vi "AO Post Step Type.vi"(8 "error in (no error)":errorcluster, 9 "AOWrite":T1, 10 "Socket No":u16=1, 11 "AO in":refnum<class "AO.lvclass">) -> (0 "error out":errorcluster, 2 "PhysicalChannel":string[](array[string]), 3 "AO out":refnum<class "AO.lvclass">)   [LabVIEW 2023, in "HardwareAbstractionLayer_LVOOP.lvlib" / "AO.lvclass"]
uses:
  AO.lvclass
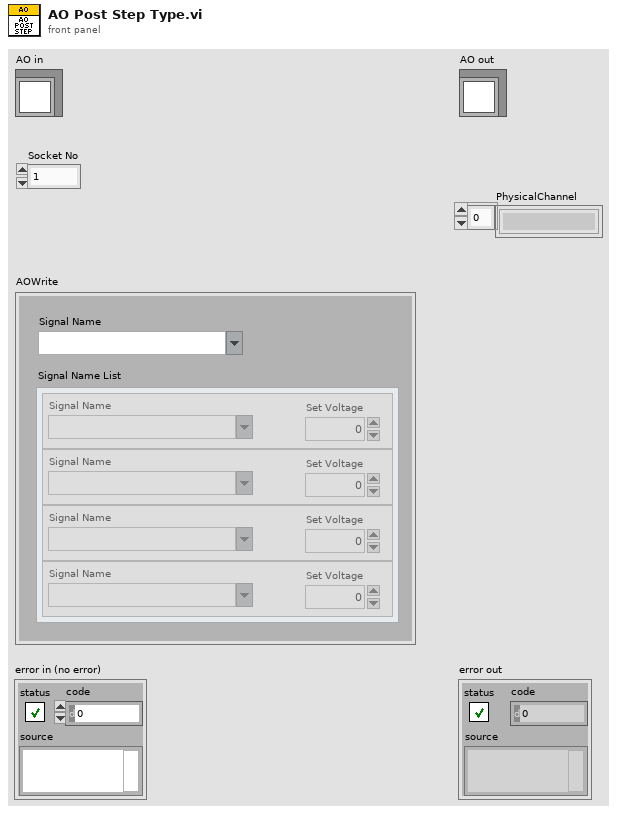
[diagram p1: front panel]
types:
  T1 = cluster{"Signal Name":string, "Signal Name List":cluster{"Signal Name":string, "Set Voltage":dbl}[]}
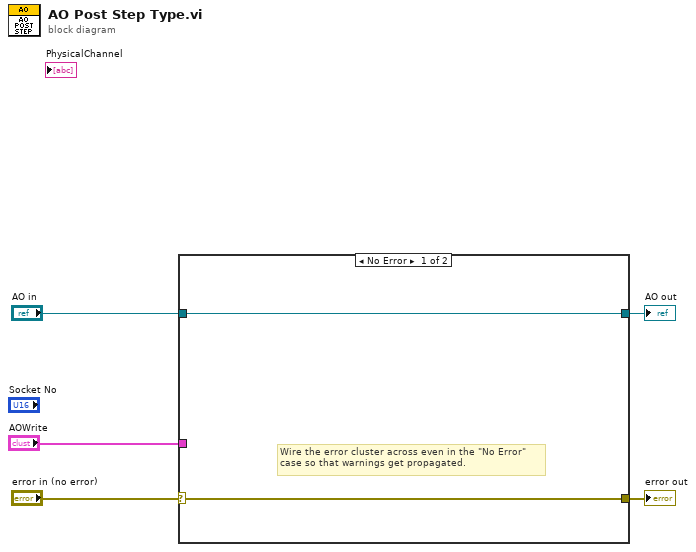
[diagram p0: block diagram]
diagram:
  n1 = case shown="No Error" "error in (no error)" {
    selector: "error in (no error)" -> [w7 w9]
    tunnel: [w7 w9] -> w4
    tunnel: [w6 w8] -> w2
    tunnel: "AO in" -> [w6 w8]
    tunnel: "AOWrite" -> [_ _]
    frame No Error {
      # "Wire the error cluster across even in the \"No Error\"\ncase so that warnings get propagated."
    }
    frame Error {
    }
  }
  "error out" <- w4
  "AO out" <- w2
